vi "Make transition array (SubVI).vi"(1 "count array in":i32[](array[numeric])) -> (0 "Transition array out":i32[](array[numeric]))   [LabVIEW 2014]
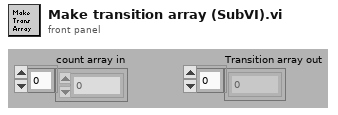
[diagram p1: front panel]
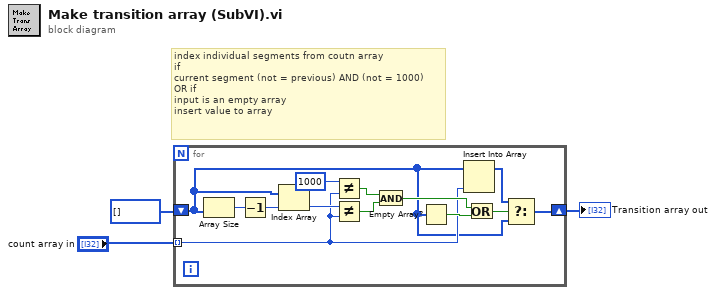
[diagram p0: block diagram]
diagram:
  # "index individual segments from coutn array\nif \ncurrent segment (not = previous) AND (not = 1000)\nOR if \ninput is an empty array \ninsert value to array"
  n1 = for {
    tunnel: "count array in" -> [w5] mode=indexing
    shift-right: [w14] -> w2
    shift-left: i32[] [] ("count array in") -> [w4]
    n2 = Array Size(array=w4) -> (size(s)=w10:i32)
    n3 = Decrement(x=w10) -> (x-1=w11:i32)
    n4 = Index Array(array=w4, index=w11) -> (element=w12:i32)
    n5 = Not Equal?(x=1000 ("y"), y=w5) -> (x != y?=w7:bool)
    n6 = Not Equal?(x=w12, y=w5) -> (x != y?=w6:bool)
    n7 = And(x=w7, y=w6) -> (x .and. y?=w9:bool)
    n8 = Empty Array?(array=w4) -> (empty?=w15:bool)
    n9 = Insert Into Array(array=w4, new element=w5) -> (w13:i32[])  [unwired: 1 in]
    n10 = Or(x=w9, y=w15) -> (x .or. y?=w16:bool)
    n11 = Select(t=w13, s=w16, f=w4) -> (s? t:f=w14:i32[])
  }
  "Transition array out" <- w2
